vi "Get Last Item on Filepath.vi"(11 "Replacement VI for SPI Engine":path) -> (3 "String":string)   [LabVIEW 2014, in "SPI Engine Scripting.lvlib"]
uses:
  SPI Engine Scripting.lvlib
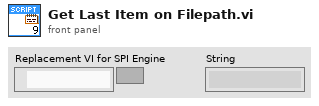
[diagram p1: front panel]
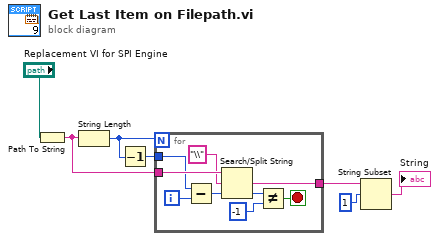
[diagram p0: block diagram]
diagram:
  n1 = Path To String(path="Replacement VI for SPI Engine") -> (string=w3:string)
  n2 = String Length(string=w3) -> (length=w2:i32)
  n3 = Decrement(x=w2) -> (x-1=w1:i32)
  n4 = for {
    N: w2 -> [_]
    tunnel: w3 -> [w16]
    tunnel: w1 -> [w11]
    tunnel: [w9] -> w4
    i -> [w10]
    stop <- w13 stop-if-true
    n5 = Subtract(x=w11, y=w10) -> (x-y=w12:i32)
    n6 = Search/Split String(string=w16, search string/char (-)="\\", offset (0)=w12) -> (match + rest of string=w9:string, offset of match=w15:i32)  [unwired: 1 out]
    n7 = Not Equal?(x=w15, y=-1) -> (x != y?=w13:bool)
  }
  n8 = String Subset(string=w4, offset (0)=1) -> (substring=→"String":string)  [unwired: 1 in]
